vi "Dust Type Updater.vi"() -> ()   [LabVIEW 2013]
uses:
  <vilib>/Utility/miscctls.llb/LVPointTypeDef.ctl
  <vilib>/addons/database/Connection.llb/Conn Execute.vi
  <vilib>/addons/database/Recordset.llb/Rec Fetch Recordset Data (R).vi
  <vilib>/addons/database/Recordset.llb/Rec Destroy - Connection.vi
  <userlib>/_OpenG.lib/array/array.llb/Remove Duplicates from 1D Array (String)__ogtk.vi
  <userlib>/_OpenG.lib/array/array.llb/Search 1D Array (String)__ogtk.vi
  <userlib>/_OpenG.lib/array/array.llb/Index 1D Array Elements (I32)__ogtk.vi
  <userlib>/_OpenG.lib/array/array.llb/Search 1D Array (I32)__ogtk.vi
  <userlib>/_OpenG.lib/array/array.llb/Filter 1D Array (I32)__ogtk.vi
  <userlib>/_OpenG.lib/array/array.llb/Conditional Auto-Indexing Tunnel (I32)__ogtk.vi
  <userlib>/_OpenG.lib/comparison/comparison.llb/Boolean Changed__ogtk.vi
  <userlib>/_OpenG.lib/comparison/comparison.llb/String Changed__ogtk.vi
  <userlib>/_OpenG.lib/comparison/comparison.llb/U16 Changed__ogtk.vi
  <userlib>/_OpenG.lib/array/array.llb/Index 1D Array Elements (DBL)__ogtk.vi
  <vilib>/addons/database/_DB Variant To Data/Database Variant To Data.xnode
  <vilib>/addons/database/NI_Database_API.lvlib
panel:
  in  "Clear Errors?":bool
  out "Shoots":bool[](array[boolean])
  in  "Change Everything":bool
  in  "New Dust":T1 {"New Batch" min=1 max=3 step=1; "New Type" min=1 max=11 step=1}
  out "Bottle Weights":dbl[](array[numeric])
  in  "Updateable Properties":T2
  in  "Create New Entry":bool
  in  "Cancel":bool
  in  "Update":bool
  in  "Update current entry":bool
  out "error IO":errorcluster
  in  "stop":bool
  out "Comments":string[](array[string])
  out "Dust Names":string[](array[string])
  out "Dust Weights":dbl[](array[numeric])
  out "Sizes":string[](array[string])
  out "Typical Weights":dbl[](array[numeric])
  out "Densities":dbl[](array[numeric])
  out "Batch Nos":i32[](array[numeric])
  out "Dust Type":i32[](array[numeric])
  out "Dust Type Ids":i32[](array[numeric])
  out "Dust Properties":T3
  in  "Dust":T4 {"Batch" min=1 max=3 step=1; "Type" min=1 max=10 step=1}
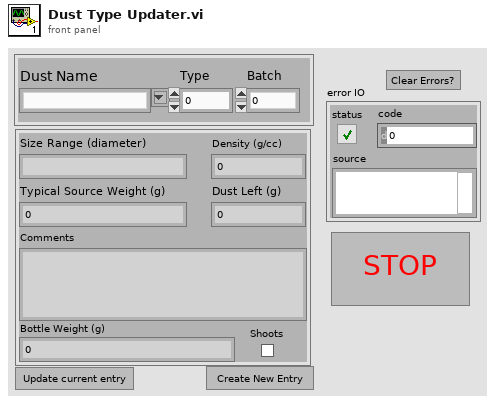
[diagram p1: front panel]
types:
  T1 = cluster{"New Dust Name":string, "New Type":u16, "New Batch":u16, "dust type id":u16, "Dust Left (g)":dbl, "Typical Source Weight (g)":dbl, "Density (g/cc)":dbl, "Size Range (diameter)":string, "Comments":string, "Bottle Weight (g)":dbl, "Shoots":bool}
  T2 = cluster{"Size Range (diameter)":string, "Density (g/cc)":dbl, "Typical Source Weight (g)":dbl, "Total Weight (g)":dbl, "Comments":string, "Bottle Weight (g)":dbl, "Shoots":bool}
  T3 = cluster{"Size Range (diameter)":string, "Density (g/cc)":dbl, "Typical Source Weight (g)":dbl, "Dust Left (g)":dbl, "Comments":string, "Bottle Weight (g)":dbl, "Shoots":bool}
  T4 = cluster{"Dust Name":string, "Type":u16, "Batch":u16, "dust type id":u16}
  T5 = typedef "LVPointTypeDef.ctl" = cluster{"Horizontal":i16, "Vertical":i16}
  T6 = enum8{"Enabled", "Disabled", "Disabled and Grayed Out"}
  T7 = typedef "NI_Database_API.lvlib/Conn ObjectReference.ctl" = refnum<k1>
  T8 = typedef "NI_Database_API.lvlib/Rec ObjectReference.ctl" = refnum<k1>
  T9 = cluster{"data":string, "data":dbl, "data":dbl, "data":dbl, "data":string, "data":dbl, "data":bool}
  T10 = cluster{"data":string, "data":dbl, "data":dbl, dbl, "data":string, "data":dbl, "data":bool}
  T11 = cluster{"Size Range (diameter)":string, "Density (g/cc)":dbl, "Typical Source Weight (g)":dbl, dbl, "Comments":string, "Bottle Weight (g)":dbl, "Shoots":bool}
  T12 = cluster{"Density (g/cc)":dbl, "Typical Source Weight (g)":dbl, "Size Range (diameter)":string, "Bottle Weight (g)":dbl, dbl, "Comments":string, i16}
  T13 = cluster{"dust type id":u16, "trimmed string":string, "New Type":u16, "New Batch":u16, "Density (g/cc)":dbl, "Typical Source Weight (g)":dbl, "Size Range (diameter)":string, "Bottle Weight (g)":dbl, "Dust Left (g)":dbl, "Comments":string, "Shoots":bool}
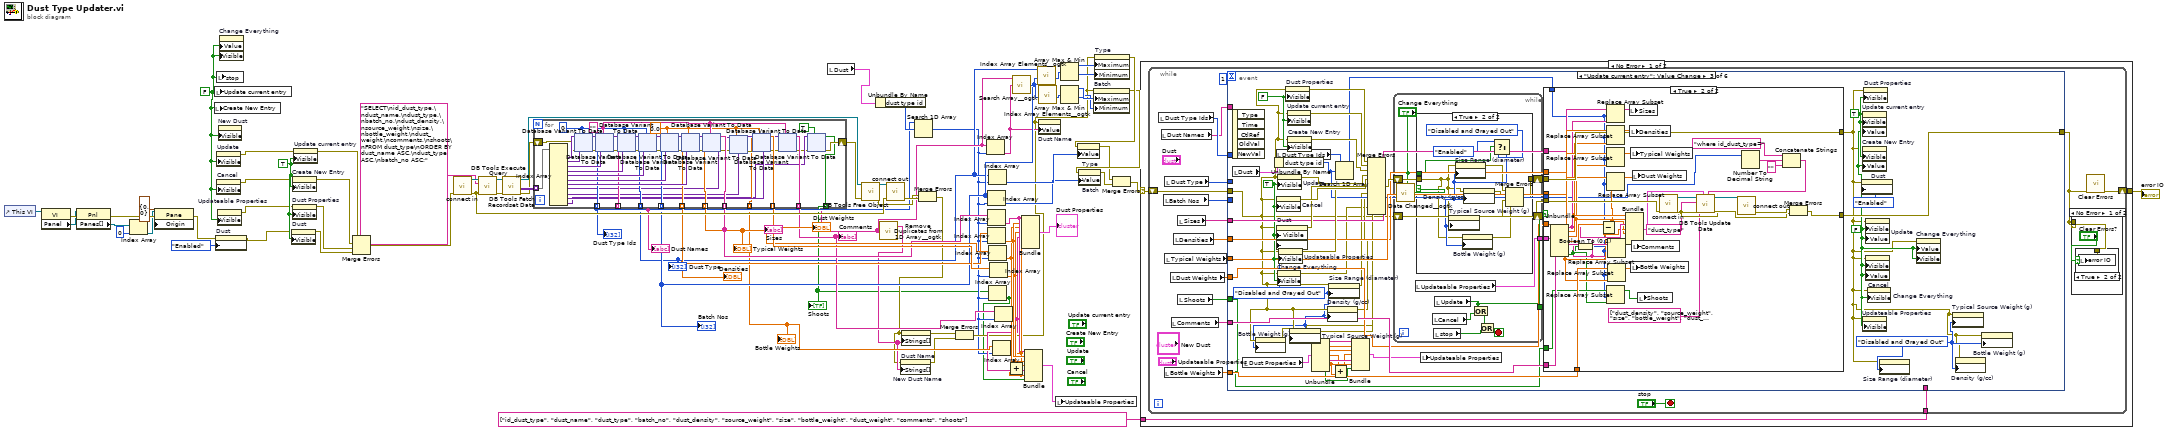
[diagram p0: block diagram]
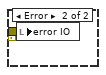
[diagram p3: hidden frame]
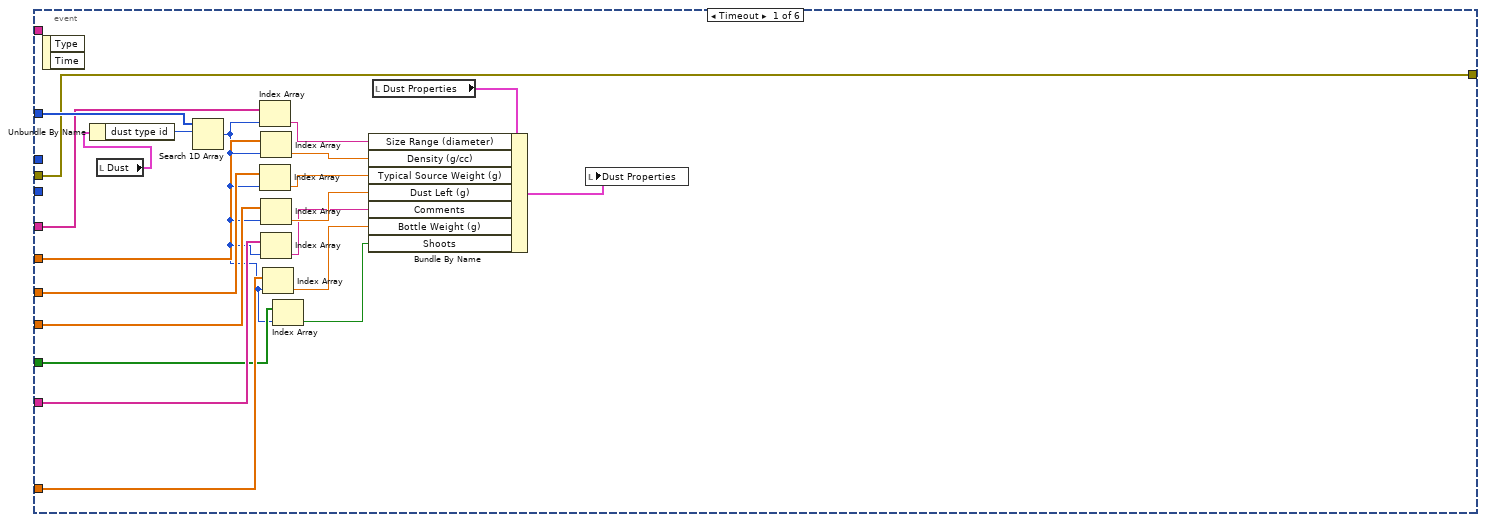
[diagram p4: hidden frame]
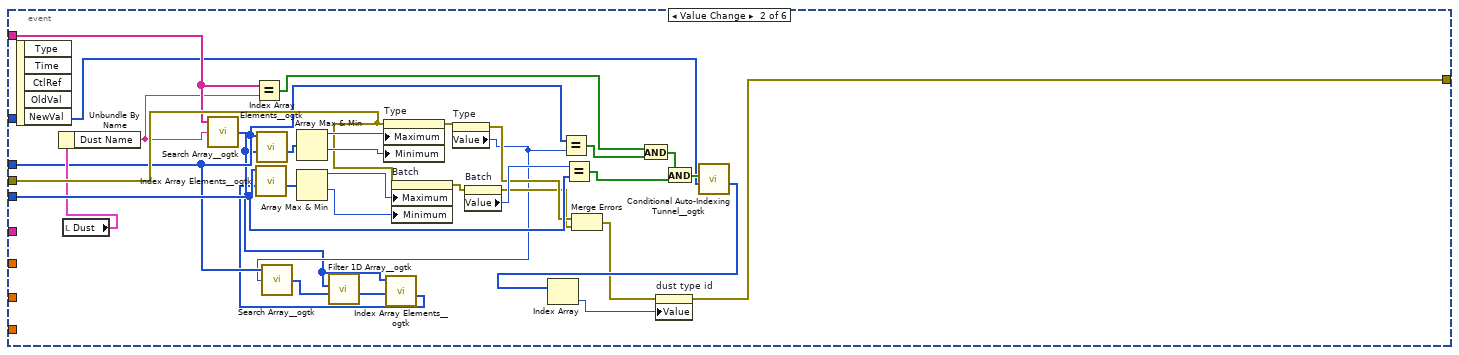
[diagram p5: hidden frame]
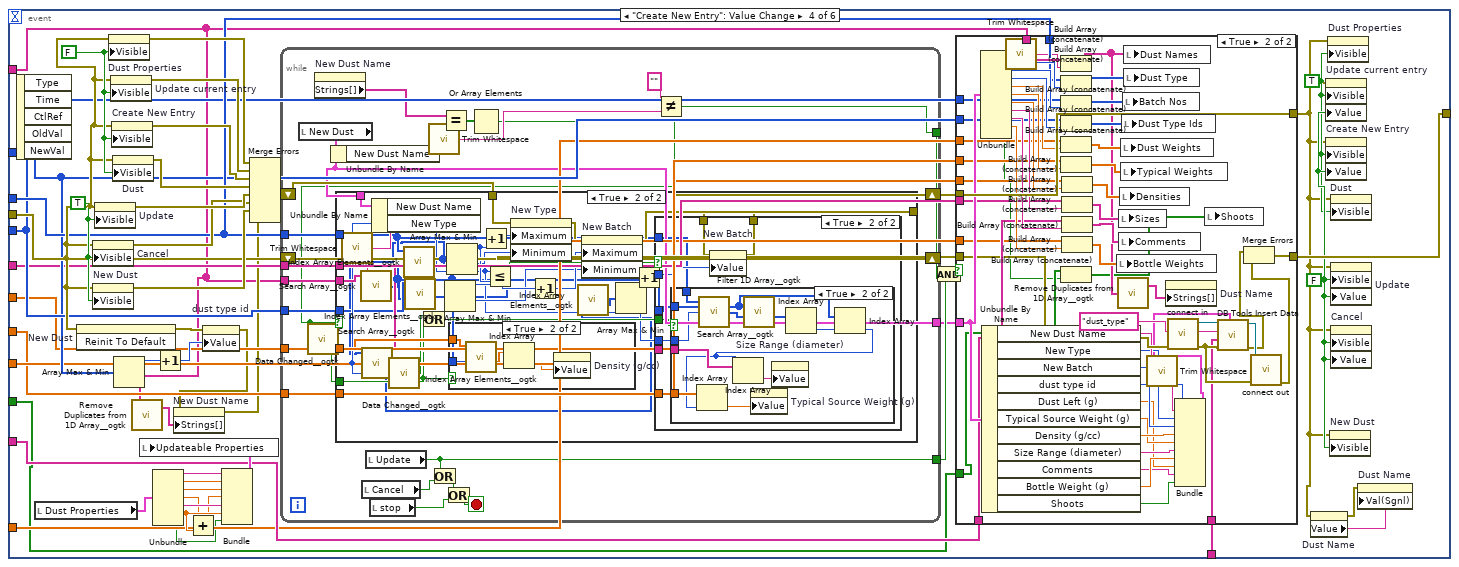
[diagram p8: hidden frame]
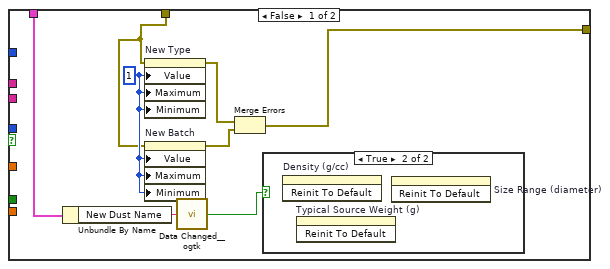
[diagram p10: hidden frame]
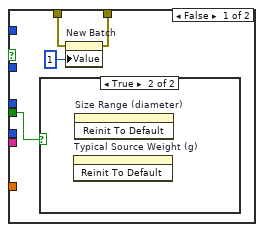
[diagram p13: hidden frame]
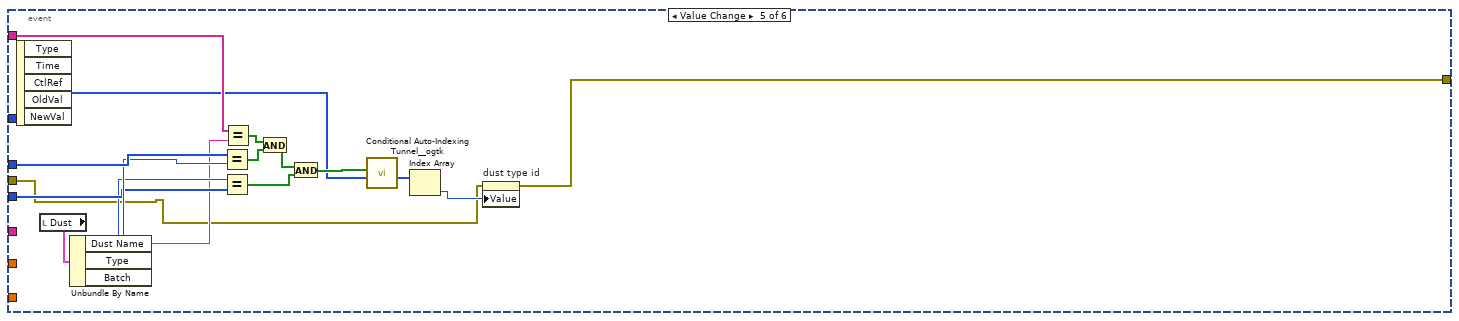
[diagram p16: hidden frame]
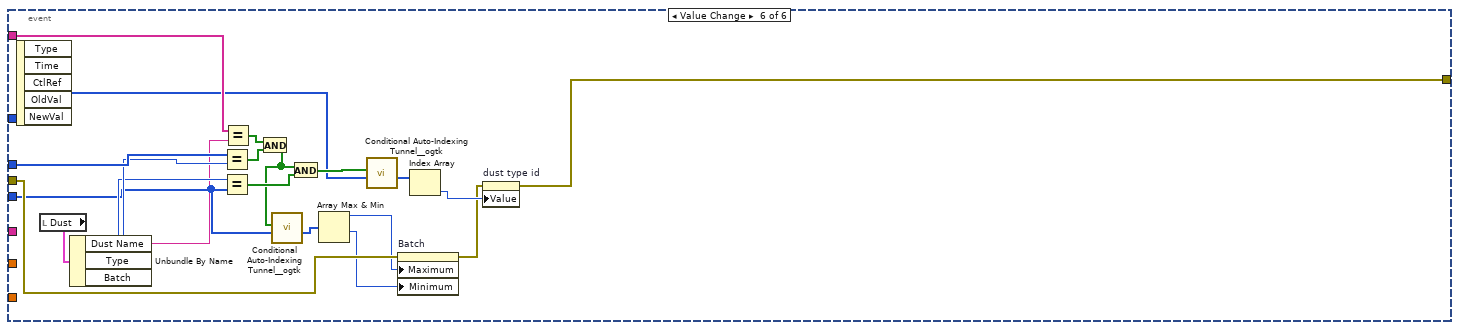
[diagram p17: hidden frame]
diagram:
  w40 = TRUE ("Visible")
  w13 = FALSE ("Update current entry")
  n1 = control-ref of="This VI"() -> (w9:refnum<vi>)
  n2 = property class="VI"(reference=w9) -> (error out=w8:errorcluster, "Panel"=w7:refnum<vi>)  [unwired: 1 in, 1 out]
  n3 = property class="Pnl"(reference=w7, error in=w8) -> (error out=w6:errorcluster, "Panes[]"=w5:refnum<vi>[])  [unwired: 1 out]
  n4 = Index Array(array=w5, index=0) -> (element=w3:refnum<vi>)
  n5 = property class="Pane"(reference=w3, error in=w6, "Origin"=T5 {"Horizontal"=0, "Vertical"=0}) -> (error out=w1:errorcluster)  [unwired: 1 out]
  n6 = local write "Create New Entry"(w13) -> ()
  n7 = local write "Update current entry"(w13) -> ()
  n8 = property on="Dust" class="Clust (strict)"(error in=w1, "DisabledEnum"=T6."Enabled" ("Disabled")) -> (error out=w31:errorcluster)  [unwired: 1 in, 1 out]
  n9 = local write "stop"(w13) -> ()
  n10 = property on="Update" class="Bool (strict)"("Visible"=w13) -> (error out=w37:errorcluster)  [unwired: 2 in, 1 out]
  n11 = property on="Cancel" class="Bool (strict)"("Visible"=w13) -> (error out=w38:errorcluster)  [unwired: 2 in, 1 out]
  n12 = property on="Updateable Properties" class="Clust (strict)"("Visible"=w13) -> (error out=w39:errorcluster)  [unwired: 2 in, 1 out]
  n13 = property on="New Dust" class="Clust (strict)"("Visible"=w13) -> ()  [unwired: 2 in, 2 out]
  n14 = property on="Change Everything" class="Bool (strict)"("Value"=w13, "Visible"=w13) -> ()  [unwired: 2 in, 2 out]
  n15 = property on="Dust" class="Clust (strict)"(error in=w31, "Visible"=w40) -> (error out=w32:errorcluster)  [unwired: 1 in, 1 out]
  n16 = property on="Create New Entry" class="Bool (strict)"(error in=w38, "Visible"=w40) -> (error out=w34:errorcluster)  [unwired: 1 in, 1 out]
  n17 = property on="Dust Properties" class="Clust (strict)"(error in=w39, "Visible"=w40) -> (error out=w33:errorcluster)  [unwired: 1 in, 1 out]
  n18 = property on="Update current entry" class="Bool (strict)"(error in=w37, "Visible"=w40) -> (error out=w35:errorcluster)  [unwired: 1 in, 1 out]
  n19 = Merge Errors(w35, w34, w33, w32) -> (w36:errorcluster)
  n20 = call <userlib>:"connect in.vi"("error in (no error)"=w36) -> ("error out"=w70:errorcluster, "Database Connection"=w77:T7)  [unwired: 7 in]
  n21 = call-poly <vilib>:"DB Tools Execute Query.vi"("error in (no error)"=w70, "SQL query"="SELECT\nid_dust_type,\ndust_name,\ndust_type,\nbatch_no,\ndust_density,\nsource_weight,\nsize,\nbottle_weight,\ndust_weight,\ncomments,\nshoots\nFROM dust_type\nORDER BY dust_name ASC,\ndust_type ASC,\nbatch_no ASC;", "connection reference"=w77) -> ("error out"=w79:errorcluster, "recordset reference"=w78:T8)  [unwired: 5 in]
  n22 = call-poly <vilib>:"DB Tools Fetch Recordset Data.vi"("error in (no error)"=w79, "recordset reference"=w78) -> ("error out"=w74:errorcluster, "recordset data"=w75:variant[][], "recordset reference out"=w71:T8)  [unwired: 3 in]
  n23 = for {
    tunnel: w75 -> [w118] mode=indexing
    shift-right: [w81] -> w72
    shift-left: w74 -> [w110]
    tunnel: [w102] -> w61 mode=indexing
    tunnel: [w101] -> w57 mode=indexing
    tunnel: [w100] -> w54 mode=indexing
    tunnel: [w99] -> w55 mode=indexing
    tunnel: [w98] -> w65 mode=indexing
    tunnel: [w97] -> w66 mode=indexing
    tunnel: [w96] -> w64 mode=indexing
    tunnel: [w95] -> w67 mode=indexing
    tunnel: [w92] -> w63 mode=indexing
    tunnel: [w85] -> w29 mode=indexing
    tunnel: [w80] -> w11 mode=indexing
    w88 = 0.0
    w94 = ""
    w103 = 0
    n24 = Index Array(array=w118) -> (element #1=w117:variant, element #2=w116:variant, element #3=w115:variant, element #4=w114:variant, element #5=w113:variant, element #6=w112:variant, element #7=w111:variant, element #8=w89:variant, element #9=w90:variant, element #10=w91:variant, element #11=w84:variant)  [unwired: 11 in]
    n25 = xnode "Database Variant To Data"("database variant"=w117, "error in (no error)"=w110, "type"=w103) -> ("data"=w102:i32, "error out"=w109:errorcluster)
    n26 = xnode "Database Variant To Data"("database variant"=w116, "error in (no error)"=w109, "type"=w94) -> ("data"=w101:string, "error out"=w108:errorcluster)
    n27 = xnode "Database Variant To Data"("database variant"=w115, "error in (no error)"=w108, "type"=w103) -> ("data"=w100:i32, "error out"=w107:errorcluster)
    n28 = xnode "Database Variant To Data"("database variant"=w114, "error in (no error)"=w107, "type"=w103) -> ("data"=w99:i32, "error out"=w106:errorcluster)
    n29 = xnode "Database Variant To Data"("database variant"=w113, "error in (no error)"=w106, "type"=w88) -> ("data"=w98:dbl, "error out"=w105:errorcluster)
    n30 = xnode "Database Variant To Data"("database variant"=w112, "error in (no error)"=w105, "type"=w88) -> ("data"=w97:dbl, "error out"=w104:errorcluster)
    n31 = xnode "Database Variant To Data"("database variant"=w111, "error in (no error)"=w104, "type"=w94) -> ("data"=w96:string, "error out"=w87:errorcluster)
    n32 = xnode "Database Variant To Data"("database variant"=w89, "error in (no error)"=w87, "type"=w88) -> ("data"=w85:dbl, "error out"=w86:errorcluster)
    n33 = xnode "Database Variant To Data"("database variant"=w90, "error in (no error)"=w86, "type"=w88) -> ("data"=w95:dbl, "error out"=w93:errorcluster)
    n34 = xnode "Database Variant To Data"("database variant"=w91, "error in (no error)"=w93, "type"=w94) -> ("data"=w92:string, "error out"=w82:errorcluster)
    n35 = xnode "Database Variant To Data"("database variant"=w84, "error in (no error)"=w82, "type"=TRUE) -> ("data"=w80:bool, "error out"=w81:errorcluster)
  }
  "Dust Type Ids" <- w61
  "Dust Type" <- w54
  "Batch Nos" <- w55
  "Densities" <- w65
  "Typical Weights" <- w66
  "Sizes" <- w64
  "Dust Weights" <- w67
  "Dust Names" <- w57
  "Comments" <- w63
  "Bottle Weights" <- w29
  "Shoots" <- w11
  n36 = local read "Dust"() -> (w41:T4)
  n37 = call-poly <vilib>:"DB Tools Free Object.vi"("error in (no error)"=w72, "recordset reference"=w71) -> ("error out"=w68:errorcluster, "connection reference"=w73:T7)  [unwired: 8 in]
  n38 = Unbundle By Name(w41) -> ("dust type id"=w62:u16)
  n39 = call-poly <userlib>:"Remove Duplicates from 1D Array__ogtk.vi"("Input Array"=w57) -> ("Output Array"=w18:string[])  [unwired: 1 out]
  n40 = call <userlib>:"connect out.vi"("error in (no error)"=w70, "connection reference"=w73) -> ("error out"=w69:errorcluster)  [unwired: 9 in]
  n41 = Search 1D Array(1D array=w61, element=w62) -> (index of element=w12:i32)  [unwired: 1 in]
  n42 = Merge Errors(w68, w69) -> (w17:errorcluster)
  n43 = property on="New Dust Name" class="CmbBox"(error in=w17, "Strings[]"=w18) -> (error out=w15:errorcluster)  [unwired: 1 in, 1 out]
  n44 = property on="Dust Name" class="CmbBox"(error in=w17, "Strings[]"=w18) -> (error out=w45:errorcluster)  [unwired: 1 in, 1 out]
  n45 = Merge Errors(w45, w15) -> (w16:errorcluster)
  n46 = Index Array(array=w57, index=w12) -> (element=w19:string)
  n47 = Index Array(array=w64, index=w12) -> (element=w26:string)
  n48 = Index Array(array=w65, index=w12) -> (element=w25:dbl)
  n49 = Index Array(array=w55, index=w12) -> (element=w58:i32)
  n50 = Index Array(array=w11, index=w12) -> (element=w10:bool)
  n51 = Index Array(array=w54, index=w12) -> (element=w59:i32)
  n52 = Index Array(array=w66, index=w12) -> (element=w24:dbl)
  n53 = Index Array(array=w67, index=w12) -> (element=w23:dbl)
  n54 = Index Array(array=w29, index=w12) -> (element=w20:dbl)
  n55 = Index Array(array=w63, index=w12) -> (element=w22:string)
  n56 = Add(x=w23, y=w20) -> (x+y=w21:dbl)
  n57 = call-poly <userlib>:"Search Array__ogtk.vi"("Array"=w57, "Element Data"=w19) -> ("Indices of Elements"=w56:i32[])  [unwired: 7 in]
  n58 = Bundle("data"=w26, "data"=w25, "data"=w24, "data"=w23, "data"=w22, "data"=w20, "data"=w10) -> (→"Dust Properties":T9)  [unwired: 1 in]
  n59 = Bundle("data"=w26, "data"=w25, "data"=w24, w21, "data"=w22, "data"=w20, "data"=w10) -> (w27:T10)  [unwired: 1 in]
  n60 = call-poly <userlib>:"Index Array Elements__ogtk.vi"("indices"=w56, "array"=w54) -> ("elements"=w53:i32[])  [unwired: 9 in]
  n61 = call-poly <userlib>:"Index Array Elements__ogtk.vi"("indices"=w56, "array"=w55) -> ("elements"=w52:i32[])  [unwired: 9 in]
  n62 = property on="Dust Name" class="CmbBox"(error in=w16, "Value"=w19) -> ()  [unwired: 1 in, 2 out]
  n63 = local write "Updateable Properties"(w27) -> ()
  n64 = Array Max & Min(array=w53) -> (max value=w51:i32, min value=w50:i32)  [unwired: 2 out]
  n65 = Array Max & Min(array=w52) -> (max value=w49:i32, min value=w48:i32)  [unwired: 2 out]
  n66 = property on="Batch" class="DigNum (strict)"(error in=w16, "Maximum"=w49, "Minimum"=w48) -> (error out=w46:errorcluster)  [unwired: 1 in, 1 out]
  n67 = property on="Batch" class="DigNum (strict)"(error in=w46, "Value"=w58) -> (error out=w43:errorcluster)  [unwired: 1 in, 1 out]
  n68 = property on="Type" class="DigNum (strict)"(error in=w16, "Maximum"=w51, "Minimum"=w50) -> (error out=w47:errorcluster)  [unwired: 1 in, 1 out]
  n69 = property on="Type" class="DigNum (strict)"(error in=w47, "Value"=w59) -> (error out=w44:errorcluster)  [unwired: 1 in, 1 out]
  n70 = Merge Errors(w44, w43) -> (w42:errorcluster)
  n71 = case shown="No Error" w42 {
    selector: w42 -> [w473 w901]
    tunnel: [w472 w901] -> w60
    tunnel: string[] ["id_dust_type", "dust_name", "dust_type", "batch_no", "dust_density", "source_weight", "size", "bottle_weight", "dust_weight", "comments", "shoots"] ("columns") -> [w471 _]
    frame No Error {
      n72 = while {
        shift-right: [w479] -> w472
        shift-left: w473 -> [w483]
        tunnel: w471 -> [w476]
        stop <- "stop" stop-if-true
        n73 = local read "Dust Type Ids"() -> (w489:i32[])
        n74 = local read "Dust Names"() -> (w482:string[])
        n75 = local read "Batch Nos"() -> (w480:i32[])
        n76 = local read "Bottle Weights"() -> (w477:dbl[])
        n77 = local read "Dust Type"() -> (w481:i32[])
        n78 = local read "Typical Weights"() -> (w486:dbl[])
        n79 = local read "Dust Weights"() -> (w485:dbl[])
        n80 = local read "Comments"() -> (w484:string[])
        n81 = local read "Densities"() -> (w487:dbl[])
        n82 = local read "Sizes"() -> (w488:string[])
        n83 = local read "Shoots"() -> (w475:bool[])
        n84 = event shown="[2] \"Update current entry\": Value Change" {
          selector: _ -> [_ _ _ _ _ _]
          dyn-events: _ -> [_ _ _ _ _ _]
          timeout: 1 -> [_ _ _ _ _ _]
          tunnel: w489 -> [w514 w532 _ w679 w869 w892]
          tunnel: w488 -> [w513 _ w567 w675 _ _]
          tunnel: w487 -> [w512 _ w568 w676 _ _]
          tunnel: w486 -> [w511 _ w569 w677 _ _]
          tunnel: w485 -> [w510 _ w570 w678 _ _]
          tunnel: w484 -> [w509 _ w571 w674 _ _]
          tunnel: w483 -> [w501 w543 w557 w685 w863 w886]
          tunnel: [w501 w526 w575 w699 w866 w889] -> w474
          tunnel: w482 -> [_ w540 _ w670 w879 w900]
          tunnel: w481 -> [_ w521 _ w681 w878 w899]
          tunnel: w480 -> [_ w539 _ w680 w876 w883]
          tunnel: w477 -> [w499 _ w572 w673 _ _]
          tunnel: w476 -> [_ _ _ w668 _ _]
          tunnel: w475 -> [w497 _ w548 w662 _ _]
          event Timeout {
            n85 = event-data() -> ()  [unwired: 1 in, 2 out]
            n86 = local read "Dust"() -> (w500:T4)
            n87 = Unbundle By Name(w500) -> ("dust type id"=w515:u16)
            n88 = Search 1D Array(1D array=w514, element=w515) -> (index of element=w496:i32)  [unwired: 1 in]
            n89 = Index Array(array=w513, index=w496) -> (element=w508:string)
            n90 = Index Array(array=w511, index=w496) -> (element=w506:dbl)
            n91 = Index Array(array=w512, index=w496) -> (element=w507:dbl)
            n92 = Index Array(array=w510, index=w496) -> (element=w505:dbl)
            n93 = Index Array(array=w509, index=w496) -> (element=w504:string)
            n94 = Index Array(array=w499, index=w496) -> (element=w498:dbl)
            n95 = Index Array(array=w497, index=w496) -> (element=w495:bool)
            n96 = local read "Dust Properties"() -> (w502:T3)
            n97 = Bundle By Name(cluster=w502, "Size Range (diameter)"=w508, "Density (g/cc)"=w507, "Typical Source Weight (g)"=w506, "Dust Left (g)"=w505, "Comments"=w504, "Bottle Weight (g)"=w498, "Shoots"=w495) -> (w503:T3)
            n98 = local write "Dust Properties"(w503) -> ()
          }
          event "Dust.Dust Name": Value Change {
            n99 = event-data() -> ()  [unwired: 1 in, 5 out]
            n100 = local read "Dust"() -> (w525:T4)
            n101 = Unbundle By Name(w525) -> ("Dust Name"=w522:string)
            n102 = call-poly <userlib>:"Search Array__ogtk.vi"("Array"=w540, "Element Data"=w522) -> ("Indices of Elements"=w517:i32[])  [unwired: 7 in]
            n103 = Equal?(x=w540, y=w522) -> (x = y?=w536:bool[])
            n104 = call-poly <userlib>:"Index Array Elements__ogtk.vi"("indices"=w517, "array"=w521) -> ("elements"=w547:i32[])  [unwired: 9 in]
            n105 = Array Max & Min(array=w547) -> (max value=w545:i32, min value=w544:i32)  [unwired: 2 out]
            n106 = property on="Type" class="DigNum (strict)"(error in=w543, "Maximum"=w545, "Minimum"=w544) -> (error out=w541:errorcluster)  [unwired: 1 in, 1 out]
            n107 = property on="Type" class="DigNum (strict)"(error in=w541) -> (error out=w529:errorcluster, "Value"=w520:u16)  [unwired: 1 in, 1 out]
            n108 = call-poly <userlib>:"Search Array__ogtk.vi"("Array"=w521, "Element Data"=w520) -> ("Indices of Elements"=w519:i32[])  [unwired: 7 in]
            n109 = call-poly <userlib>:"Filter 1D Array__ogtk.vi"("items to filter"=w519, "array"=w517) -> ("filtered item indices"=w518:i32[])  [unwired: 4 in, 1 out]
            n110 = call-poly <userlib>:"Index Array Elements__ogtk.vi"("indices"=w518, "array"=w517) -> ("elements"=w516:i32[])  [unwired: 9 in]
            n111 = call-poly <userlib>:"Index Array Elements__ogtk.vi"("indices"=w516, "array"=w539) -> ("elements"=w546:i32[])  [unwired: 9 in]
            n112 = Array Max & Min(array=w546) -> (max value=w523:i32, min value=w524:i32)  [unwired: 2 out]
            n113 = property on="Batch" class="DigNum (strict)"(error in=w543, "Maximum"=w523, "Minimum"=w524) -> (error out=w542:errorcluster)  [unwired: 1 in, 1 out]
            n114 = property on="Batch" class="DigNum (strict)"(error in=w542) -> (error out=w528:errorcluster, "Value"=w538:u16)  [unwired: 1 in, 1 out]
            n115 = Equal?(x=w521, y=w520) -> (x = y?=w537:bool[])
            n116 = Equal?(x=w538, y=w539) -> (x = y?=w534:bool[])
            n117 = Merge Errors(w529, w528) -> (w527:errorcluster)
            n118 = And(x=w536, y=w537) -> (x .and. y?=w535:bool[])
            n119 = And(x=w535, y=w534) -> (x .and. y?=w533:bool[])
            n120 = call-poly <userlib>:"Conditional Auto-Indexing Tunnel__ogtk.vi"("Array in"=w532, "Elements to keep"=w533) -> ("Filtered Array out"=w531:i32[])  [unwired: 5 in]
            n121 = Index Array(array=w531) -> (element=w530:i32)  [unwired: 1 in]
            n122 = property on="dust type id" class="Ring (strict)"(error in=w527, "Value"=w530) -> (error out=w526:errorcluster)  [unwired: 1 in, 1 out]
          }
          event "Update current entry": Value Change {
            w555 = T6."Disabled and Grayed Out" ("Disabled")
            w552 = T6."Disabled and Grayed Out" ("Disabled")
            w554 = FALSE ("Visible")
            w577 = TRUE ("Visible")
            w559 = TRUE ("Visible")
            w580 = FALSE ("Update current entry")
            n123 = event-data() -> ()  [unwired: 1 in, 5 out]
            n124 = local read "Dust"() -> (w591:T4)
            n125 = local read "Dust Properties"() -> (w551:T3)
            n126 = property on="Bottle Weight (g)" class="DigNum (strict)"(error in=w557, "DisabledEnum"=w552) -> (error out=w556:errorcluster)  [unwired: 1 in, 1 out]
            n127 = Unbundle By Name(w591) -> ("dust type id"=w563:u16)
            n128 = local read "Dust Type Ids"() -> (w590:i32[])
            n129 = property on="Cancel" class="Bool (strict)"(error in=w557, "Visible"=w559) -> (error out=w586:errorcluster)  [unwired: 1 in, 1 out]
            n130 = property on="Dust" class="Clust (strict)"(error in=w557, "Visible"=w559, "DisabledEnum"=w552) -> (error out=w585:errorcluster)  [unwired: 1 in, 1 out]
            n131 = property on="Change Everything" class="Bool (strict)"(error in=w557, "Visible"=w559) -> (error out=w558:errorcluster)  [unwired: 1 in, 1 out]
            n132 = property on="Update" class="Bool (strict)"(error in=w557, "Visible"=w559) -> (error out=w587:errorcluster)  [unwired: 1 in, 1 out]
            n133 = property on="Updateable Properties" class="Clust (strict)"(error in=w557, "Visible"=w559) -> (error out=w584:errorcluster)  [unwired: 1 in, 1 out]
            n134 = property on="Dust Properties" class="Clust (strict)"(error in=w557, "Visible"=w580) -> (error out=w579:errorcluster)  [unwired: 1 in, 1 out]
            n135 = property on="Update current entry" class="Bool (strict)"(error in=w557, "Visible"=w580) -> (error out=w589:errorcluster)  [unwired: 1 in, 1 out]
            n136 = property on="Create New Entry" class="Bool (strict)"(error in=w557, "Visible"=w580) -> (error out=w588:errorcluster)  [unwired: 1 in, 1 out]
            n137 = property on="Typical Source Weight (g)" class="DigNum (strict)"(error in=w557, "DisabledEnum"=w552) -> (error out=w560:errorcluster)  [unwired: 1 in, 1 out]
            n138 = Unbundle(w551) -> ("Size Range (diameter)"=w595:string, "Density (g/cc)"=w594:dbl, "Typical Source Weight (g)"=w593:dbl, "Dust Left (g)"=w565:dbl, "Comments"=w592:string, "Bottle Weight (g)"=w566:dbl, "Shoots"=w549:bool)
            n139 = property on="Density (g/cc)" class="DigNum (strict)"(error in=w557, "DisabledEnum"=w552) -> (error out=w561:errorcluster)  [unwired: 1 in, 1 out]
            n140 = property on="Size Range (diameter)" class="Str"(error in=w557, "DisabledEnum"=w552) -> (error out=w562:errorcluster)  [unwired: 1 in, 1 out]
            n141 = Add(x=w565, y=w566) -> (x+y=w564:dbl)
            n142 = Search 1D Array(1D array=w590, element=w563) -> (index of element=w574:i32)  [unwired: 1 in]
            n143 = Bundle("Size Range (diameter)"=w595, "Density (g/cc)"=w594, "Typical Source Weight (g)"=w593, w564, "Comments"=w592, "Bottle Weight (g)"=w566, "Shoots"=w549) -> (w550:T11)  [unwired: 1 in]
            n144 = Merge Errors(w579, w589, w588, w587, w586, w585, w584, w562, w561, w560, w558, w556) -> (w583:errorcluster)
            n145 = while {
              shift-right: [w639] -> w581
              shift-left: w583 -> [w643]
              tunnel: [w649] -> w573
              tunnel: [w647] -> w582
              shift-right: [w642] -> w576
              shift-left: w557 -> [w642]
              stop <- w645 stop-if-true
              n146 = call-poly <userlib>:"Data Changed__ogtk.vi"("Boolean"="Change Everything") -> ("Changed"=w641:bool)
              n147 = local read "Updateable Properties"() -> (w649:T2)
              n148 = case shown="True" w641 {
                tunnel: w643 -> [w650 w656]
                tunnel: "Change Everything" -> [_ w660]
                tunnel: [w650 w651] -> w639
                frame False {
                }
                frame True {
                  n149 = Select(t=T6."Enabled" ("Disabled"), s=w660, f=T6."Disabled and Grayed Out" ("Disabled")) -> (s? t:f=w657:T6)
                  n150 = property on="Typical Source Weight (g)" class="DigNum (strict)"(error in=w656, "DisabledEnum"=w657) -> (error out=w653:errorcluster)  [unwired: 1 in, 1 out]
                  n151 = property on="Size Range (diameter)" class="Str"(error in=w656, "DisabledEnum"=w657) -> (error out=w655:errorcluster)  [unwired: 1 in, 1 out]
                  n152 = property on="Bottle Weight (g)" class="DigNum (strict)"(error in=w656, "DisabledEnum"=w657) -> (error out=w652:errorcluster)  [unwired: 1 in, 1 out]
                  n153 = property on="Density (g/cc)" class="DigNum (strict)"(error in=w656, "DisabledEnum"=w657) -> (error out=w654:errorcluster)  [unwired: 1 in, 1 out]
                  n154 = Merge Errors(w655, w654, w653, w652) -> (w651:errorcluster)
                }
              }
              n155 = local read "Cancel"() -> (w646:bool)
              n156 = local read "stop"() -> (w644:bool)
              n157 = local read "Update"() -> (w647:bool)
              n158 = Or(x=w647, y=w646) -> (x .or. y?=w648:bool)
              n159 = Or(x=w648, y=w644) -> (x .or. y?=w645:bool)
            }
            n160 = local write "Updateable Properties"(w550) -> ()
            n161 = case shown="True" w582 {
              tunnel: w581 -> [w597 w638]
              tunnel: [w597 w638] -> w553
              tunnel: w576 -> [w596 w623]
              tunnel: [w596 w622] -> w575
              tunnel: w574 -> [_ w600]
              tunnel: w573 -> [_ w637]
              tunnel: w572 -> [_ w636]
              tunnel: w571 -> [_ w635]
              tunnel: w570 -> [_ w634]
              tunnel: w569 -> [_ w633]
              tunnel: w568 -> [_ w632]
              tunnel: w567 -> [_ w631]
              tunnel: w563 -> [_ w603]
              tunnel: w548 -> [_ w601]
              frame False {
              }
              frame True {
                n162 = Unbundle(w637) -> ("Size Range (diameter)"=w608:string, "Density (g/cc)"=w610:dbl, "Typical Source Weight (g)"=w609:dbl, "Total Weight (g)"=w624:dbl, "Comments"=w605:string, "Bottle Weight (g)"=w607:dbl, "Shoots"=w599:bool)
                n163 = Boolean To (0,1)(Boolean=w599) -> (0, 1=w602:i16)
                n164 = Subtract(x=w624, y=w607) -> (x-y=w606:dbl)
                n165 = Replace Array Subset(array=w631, new element=w608, index=w600) -> (w630:string[])
                n166 = Replace Array Subset(array=w632, new element=w610, index=w600) -> (w629:dbl[])
                n167 = Replace Array Subset(array=w633, new element=w609, index=w600) -> (w628:dbl[])
                n168 = Replace Array Subset(array=w634, new element=w606, index=w600) -> (w627:dbl[])
                n169 = Replace Array Subset(array=w601, new element=w599, index=w600) -> (w598:bool[])
                n170 = Replace Array Subset(array=w636, new element=w607, index=w600) -> (w626:dbl[])
                n171 = Replace Array Subset(array=w635, new element=w605, index=w600) -> (w625:string[])
                n172 = Bundle("Density (g/cc)"=w610, "Typical Source Weight (g)"=w609, "Size Range (diameter)"=w608, "Bottle Weight (g)"=w607, w606, "Comments"=w605, w602) -> (w604:T12)  [unwired: 1 in]
                n173 = local write "Sizes"(w630) -> ()
                n174 = local write "Densities"(w629) -> ()
                n175 = local write "Typical Weights"(w628) -> ()
                n176 = local write "Bottle Weights"(w626) -> ()
                n177 = local write "Comments"(w625) -> ()
                n178 = local write "Dust Weights"(w627) -> ()
                n179 = local write "Shoots"(w598) -> ()
                n180 = call <userlib>:"connect in.vi"("error in (no error)"=w623) -> ("error out"=w619:errorcluster, "Database Connection"=w617:T7)  [unwired: 7 in]
                n181 = Number To Decimal String(number=w603) -> (decimal integer string=w613:string)  [unwired: 1 in]
                n182 = Concatenate Strings("where id_dust_type=" ("condition"), w613, "" ("string")) -> (w611:string)
                n183 = call <vilib>:"DB Tools Update Data.vi"("condition"=w611, "data"=w604, "error in (no error)"=w619, "columns"=string[] ["dust_density", "source_weight", "size", "bottle_weight", "dust_weight", "comments", "shoots"], "table"="dust_type", "connection reference"=w617) -> ("error out"=w620:errorcluster, "connection reference out"=w616:T7)  [unwired: 4 in]
                n184 = call <userlib>:"connect out.vi"("error in (no error)"=w619, "connection reference"=w616) -> ("error out"=w621:errorcluster)  [unwired: 9 in]
                n185 = Merge Errors(w621, w620) -> (w622:errorcluster)
              }
            }
            n186 = property on="Dust" class="Clust (strict)"(error in=w553, "DisabledEnum"=T6."Enabled" ("Disabled")) -> ()  [unwired: 1 in, 2 out]
            n187 = property on="Update current entry" class="Bool (strict)"(error in=w553, "Visible"=w577, "Value"=w554) -> ()  [unwired: 1 in, 2 out]
            n188 = property on="Create New Entry" class="Bool (strict)"(error in=w553, "Visible"=w577, "Value"=w554) -> ()  [unwired: 1 in, 2 out]
            n189 = property on="Updateable Properties" class="Clust (strict)"(error in=w553, "Visible"=w554) -> ()  [unwired: 1 in, 2 out]
            n190 = property on="Dust Properties" class="Clust (strict)"(error in=w553, "Visible"=w577) -> ()  [unwired: 1 in, 2 out]
            n191 = property on="Update" class="Bool (strict)"(error in=w553, "Visible"=w554, "Value"=w554) -> ()  [unwired: 1 in, 2 out]
            n192 = property on="Cancel" class="Bool (strict)"(error in=w553, "Visible"=w554, "Value"=w554) -> ()  [unwired: 1 in, 2 out]
            n193 = property on="Change Everything" class="Bool (strict)"(error in=w553, "Visible"=w554) -> ()  [unwired: 1 in, 2 out]
            n194 = property on="Size Range (diameter)" class="Str"(error in=w553, "DisabledEnum"=w555) -> ()  [unwired: 1 in, 2 out]
            n195 = property on="Change Everything" class="Bool (strict)"(error in=w553, "Value"=w554, "Visible"=w554) -> ()  [unwired: 1 in, 2 out]
            n196 = property on="Typical Source Weight (g)" class="DigNum (strict)"(error in=w553, "DisabledEnum"=w555) -> ()  [unwired: 1 in, 2 out]
            n197 = property on="Density (g/cc)" class="DigNum (strict)"(error in=w553, "DisabledEnum"=w555) -> ()  [unwired: 1 in, 2 out]
            n198 = property on="Bottle Weight (g)" class="DigNum (strict)"(error in=w553, "DisabledEnum"=w555) -> ()  [unwired: 1 in, 2 out]
          }
          event "Create New Entry": Value Change {
            w688 = FALSE ("Visible")
            w687 = TRUE ("Visible")
            w693 = TRUE ("Visible")
            w694 = FALSE ("Update current entry")
            n199 = event-data() -> ()  [unwired: 1 in, 5 out]
            n200 = local read "Dust Properties"() -> (w711:T3)
            n201 = invoke on="New Dust" class="Clust (strict)" method="Reinit To Default"(error in=w685) -> (error out=w684:errorcluster)  [unwired: 2 in, 2 out]
            n202 = property on="Cancel" class="Bool (strict)"(error in=w685, "Visible"=w693) -> (error out=w690:errorcluster)  [unwired: 1 in, 1 out]
            n203 = property on="New Dust" class="Clust (strict)"(error in=w685, "Visible"=w693) -> (error out=w689:errorcluster)  [unwired: 1 in, 1 out]
            n204 = property on="Update" class="Bool (strict)"(error in=w685, "Visible"=w693) -> (error out=w691:errorcluster)  [unwired: 1 in, 1 out]
            n205 = property on="Dust Properties" class="Clust (strict)"(error in=w685, "Visible"=w694) -> (error out=w701:errorcluster)  [unwired: 1 in, 1 out]
            n206 = property on="Update current entry" class="Bool (strict)"(error in=w685, "Visible"=w694) -> (error out=w706:errorcluster)  [unwired: 1 in, 1 out]
            n207 = property on="Create New Entry" class="Bool (strict)"(error in=w685, "Visible"=w694) -> (error out=w705:errorcluster)  [unwired: 1 in, 1 out]
            n208 = property on="Dust" class="Clust (strict)"(error in=w685, "Visible"=w694) -> (error out=w692:errorcluster)  [unwired: 1 in, 1 out]
            n209 = Array Max & Min(array=w679) -> (max value=w683:i32)  [unwired: 3 out]
            n210 = call-poly <userlib>:"Remove Duplicates from 1D Array__ogtk.vi"("Input Array"=w670) -> ("Output Array"=w669:string[])  [unwired: 1 out]
            n211 = Unbundle(w711) -> ("Size Range (diameter)"=w710:string, "Density (g/cc)"=w709:dbl, "Typical Source Weight (g)"=w708:dbl, "Dust Left (g)"=w696:dbl, "Comments"=w707:string, "Bottle Weight (g)"=w697:dbl, "Shoots"=w661:bool)
            n212 = Increment(x=w683) -> (x+1=w682:i32)
            n213 = Add(x=w696, y=w697) -> (x+y=w695:dbl)
            n214 = property on="dust type id" class="DigNum (strict)"(error in=w684, "Value"=w682) -> (error out=w672:errorcluster)  [unwired: 1 in, 1 out]
            n215 = property on="New Dust Name" class="CmbBox"(error in=w672, "Strings[]"=w669) -> (error out=w671:errorcluster)  [unwired: 1 in, 1 out]
            n216 = Bundle("Size Range (diameter)"=w710, "Density (g/cc)"=w709, "Typical Source Weight (g)"=w708, w695, "Comments"=w707, "Bottle Weight (g)"=w697, "Shoots"=w661) -> (w698:T11)  [unwired: 1 in]
            n217 = local write "Updateable Properties"(w698) -> ()
            n218 = Merge Errors(w701, w706, w705, w692, w691, w690, w689, w671) -> (w704:errorcluster)
            n219 = while {
              shift-right: [w782] -> w702
              shift-left: w704 -> [w783]
              tunnel: [w792] -> w703
              shift-right: [w793] -> w700
              shift-left: w685 -> [w793]
              tunnel: [w780] -> w686
              tunnel: w670 -> [w786]
              tunnel: w680 -> [w785]
              tunnel: w681 -> [w784]
              tunnel: w676 -> [w781]
              tunnel: w675 -> [w779]
              tunnel: w677 -> [w778]
              tunnel: [w776] -> w666
              stop <- w791 stop-if-true
              n220 = local read "New Dust"() -> (w780:T1)
              n221 = property on="New Dust Name" class="CmbBox"() -> ("Strings[]"=w789:string[])  [unwired: 2 in, 2 out]
              n222 = Unbundle By Name(w780) -> ("New Dust Name"=w787:string)
              n223 = local read "Cancel"() -> (w795:bool)
              n224 = local read "Update"() -> (w792:bool)
              n225 = local read "stop"() -> (w790:bool)
              n226 = call <vilib>:"Trim Whitespace.vi"("string"=w787) -> ("trimmed string"=w775:string)  [unwired: 1 in]
              n227 = Or(x=w792, y=w795) -> (x .or. y?=w794:bool)
              n228 = Equal?(x=w789, y=w775) -> (x = y?=w788:bool[])
              n229 = Or(x=w794, y=w790) -> (x .or. y?=w791:bool)
              n230 = Or Array Elements(Boolean array=w788) -> (logical OR=w774:bool)
              n231 = call-poly <userlib>:"Data Changed__ogtk.vi"("Boolean"=w774) -> ("Changed"=w773:bool)
              n232 = case shown="True" w774 {
                tunnel: w786 -> [_ w834]
                tunnel: w785 -> [_ w811]
                tunnel: w784 -> [_ w813]
                tunnel: w783 -> [w802 w830]
                tunnel: [w799 w831] -> w782
                tunnel: w781 -> [_ w822]
                tunnel: w780 -> [w798 w824]
                tunnel: w779 -> [_ w820]
                tunnel: w778 -> [_ w819]
                tunnel: w773 -> [_ w814]
                frame False {
                  w803 = u16 1 ("Value")
                  n233 = Unbundle By Name(w798) -> ("New Dust Name"=w797:string)
                  n234 = property on="New Type" class="DigNum (strict)"(error in=w802, "Value"=w803, "Maximum"=w803, "Minimum"=w803) -> (error out=w801:errorcluster)  [unwired: 1 in, 1 out]
                  n235 = property on="New Batch" class="DigNum (strict)"(error in=w802, "Value"=w803, "Maximum"=w803, "Minimum"=w803) -> (error out=w800:errorcluster)  [unwired: 1 in, 1 out]
                  n236 = call-poly <userlib>:"Data Changed__ogtk.vi"("String"=w797) -> ("Changed"=w796:bool)
                  n237 = Merge Errors(w801, w800) -> (w799:errorcluster)
                  n238 = case shown="True" w796 {
                    frame False {
                    }
                    frame True {
                      n239 = invoke on="Density (g/cc)" class="DigNum (strict)" method="Reinit To Default"() -> ()  [unwired: 3 in, 3 out]
                      n240 = invoke on="Typical Source Weight (g)" class="DigNum (strict)" method="Reinit To Default"() -> ()  [unwired: 3 in, 3 out]
                      n241 = invoke on="Size Range (diameter)" class="Str" method="Reinit To Default"() -> ()  [unwired: 3 in, 3 out]
                    }
                  }
                }
                frame True {
                  n242 = Unbundle By Name(w824) -> ("New Dust Name"=w823:string, "New Type"=w812:u16)
                  n243 = call <vilib>:"Trim Whitespace.vi"("string"=w823) -> ("trimmed string"=w816:string)  [unwired: 1 in]
                  n244 = call-poly <userlib>:"Search Array__ogtk.vi"("Array"=w834, "Element Data"=w816) -> ("Indices of Elements"=w808:i32[])  [unwired: 7 in]
                  n245 = call-poly <userlib>:"Data Changed__ogtk.vi"("U16"=w812) -> ("Changed"=w821:bool)
                  n246 = call-poly <userlib>:"Index Array Elements__ogtk.vi"("indices"=w808, "array"=w813) -> ("elements"=w810:i32[])  [unwired: 9 in]
                  n247 = call-poly <userlib>:"Search Array__ogtk.vi"("Array"=w810, "Element Data"=w812) -> ("Indices of Elements"=w809:i32[])  [unwired: 7 in]
                  n248 = call-poly <userlib>:"Index Array Elements__ogtk.vi"("indices"=w808, "array"=w811) -> ("elements"=w804:i32[])  [unwired: 9 in]
                  n249 = Or(x=w821, y=w814) -> (x .or. y?=w815:bool)
                  n250 = Array Max & Min(array=w804) -> (max value=w832:i32, min value=w817:i32)  [unwired: 2 out]
                  n251 = Array Max & Min(array=w810) -> (max value=w829:i32, min value=w818:i32)  [unwired: 2 out]
                  n252 = case shown="True" w814 {
                    tunnel: w822 -> [_ w837]
                    tunnel: w808 -> [_ w836]
                    frame False {
                    }
                    frame True {
                      n253 = call-poly <userlib>:"Index Array Elements__ogtk.vi"("indices"=w836, "array"=w837) -> ("elements"=w838:dbl[])  [unwired: 9 in]
                      n254 = Index Array(array=w838) -> (element=w835:dbl)  [unwired: 1 in]
                      n255 = property on="Density (g/cc)" class="DigNum (strict)"("Value"=w835) -> ()  [unwired: 2 in, 2 out]
                    }
                  }
                  n256 = Increment(x=w829) -> (x+1=w825:i32)
                  n257 = Less Or Equal?(x=w812, y=w829) -> (x <= y?=w833:bool)
                  n258 = property on="New Type" class="DigNum (strict)"(error in=w830, "Maximum"=w825, "Minimum"=w818) -> (error out=w828:errorcluster)  [unwired: 1 in, 1 out]
                  n259 = Increment(x=w832) -> (x+1=w826:i32)
                  n260 = call-poly <userlib>:"Index Array Elements__ogtk.vi"("indices"=w809, "array"=w804) -> ("elements"=w806:i32[])  [unwired: 9 in]
                  n261 = property on="New Batch" class="DigNum (strict)"(error in=w828, "Maximum"=w826, "Minimum"=w817) -> (error out=w827:errorcluster)  [unwired: 1 in, 1 out]
                  n262 = Array Max & Min(array=w806) -> (max value=w807:i32)  [unwired: 3 out]
                  n263 = Increment(x=w807) -> (x+1=w805:i32)
                  n264 = case shown="True" w833 {
                    tunnel: w805 -> [_ w851]
                    tunnel: w827 -> [w841 w850]
                    tunnel: [w840 w849] -> w831
                    tunnel: w815 -> [w839 w848]
                    tunnel: w812 -> [_ w847]
                    tunnel: w808 -> [_ w846]
                    tunnel: w813 -> [_ w845]
                    tunnel: w820 -> [_ w844]
                    tunnel: w819 -> [_ w843]
                    frame False {
                      n265 = case shown="True" w839 {
                        frame False {
                        }
                        frame True {
                          n266 = invoke on="Typical Source Weight (g)" class="DigNum (strict)" method="Reinit To Default"() -> ()  [unwired: 3 in, 3 out]
                          n267 = invoke on="Size Range (diameter)" class="Str" method="Reinit To Default"() -> ()  [unwired: 3 in, 3 out]
                        }
                      }
                      n268 = property on="New Batch" class="DigNum (strict)"(error in=w841, "Value"=u16 1) -> (error out=w840:errorcluster)  [unwired: 1 in, 1 out]
                    }
                    frame True {
                      n269 = case shown="True" w848 {
                        tunnel: w847 -> [_ w861]
                        tunnel: w846 -> [_ w853]
                        tunnel: w845 -> [_ w862]
                        tunnel: w844 -> [_ w859]
                        tunnel: w843 -> [_ w858]
                        frame False {
                        }
                        frame True {
                          n270 = call-poly <userlib>:"Search Array__ogtk.vi"("Array"=w862, "Element Data"=w861) -> ("Indices of Elements"=w860:i32[])  [unwired: 7 in]
                          n271 = call-poly <userlib>:"Filter 1D Array__ogtk.vi"("items to filter"=w860, "array"=w853) -> ("filtered item indices"=w855:i32[])  [unwired: 4 in, 1 out]
                          n272 = Index Array(array=w855) -> (element=w854:i32)  [unwired: 1 in]
                          n273 = Index Array(array=w853, index=w854) -> (element=w852:i32)
                          n274 = Index Array(array=w858, index=w852) -> (element=w856:dbl)
                          n275 = Index Array(array=w859, index=w852) -> (element=w857:string)
                          n276 = property on="Typical Source Weight (g)" class="DigNum (strict)"("Value"=w856) -> ()  [unwired: 2 in, 2 out]
                          n277 = property on="Size Range (diameter)" class="Str"("Value"=w857) -> ()  [unwired: 2 in, 2 out]
                        }
                      }
                      n278 = property on="New Batch" class="DigNum (strict)"(error in=w850, "Value"=w851) -> (error out=w849:errorcluster)  [unwired: 1 in, 1 out]
                    }
                  }
                }
              }
              n279 = Not Equal?(x="", y=w775) -> (x != y?=w776:bool)
            }
            n280 = And(x=w703, y=w666) -> (x .and. y?=w667:bool)
            n281 = case shown="True" w667 {
              tunnel: w702 -> [w713 w772]
              tunnel: [w713 w772] -> w664
              tunnel: w700 -> [w712 w738]
              tunnel: [w712 w722] -> w699
              tunnel: w686 -> [_ w771]
              tunnel: w670 -> [_ w760]
              tunnel: w681 -> [_ w759]
              tunnel: w680 -> [_ w758]
              tunnel: w679 -> [_ w757]
              tunnel: w678 -> [_ w756]
              tunnel: w677 -> [_ w755]
              tunnel: w676 -> [_ w754]
              tunnel: w675 -> [_ w753]
              tunnel: w674 -> [_ w752]
              tunnel: w673 -> [_ w751]
              tunnel: w668 -> [_ w736]
              tunnel: w662 -> [_ w717]
              frame False {
              }
              frame True {
                n282 = Unbundle(w771) -> ("New Dust Name"=w770:string, "New Type"=w769:u16, "New Batch"=w768:u16, "dust type id"=w767:u16, "Dust Left (g)"=w766:dbl, "Typical Source Weight (g)"=w765:dbl, "Density (g/cc)"=w764:dbl, "Size Range (diameter)"=w763:string, "Comments"=w762:string, "Bottle Weight (g)"=w761:dbl, "Shoots"=w716:bool)
                n283 = Unbundle By Name(w771) -> ("New Dust Name"=w732:string, "New Type"=w731:u16, "New Batch"=w730:u16, "dust type id"=w733:u16, "Dust Left (g)"=w725:dbl, "Typical Source Weight (g)"=w728:dbl, "Density (g/cc)"=w729:dbl, "Size Range (diameter)"=w727:string, "Comments"=w724:string, "Bottle Weight (g)"=w726:dbl, "Shoots"=w714:bool)
                n284 = call <vilib>:"Trim Whitespace.vi"("string"=w770) -> ("trimmed string"=w719:string)  [unwired: 1 in]
                n285 = Build Array (concatenate)(w760, w719) -> (w741:string[])
                n286 = Build Array (concatenate)(w759, w769) -> (w750:i32[])
                n287 = Build Array (concatenate)(w758, w768) -> (w749:i32[])
                n288 = Build Array (concatenate)(w757, w767) -> (w748:i32[])
                n289 = Build Array (concatenate)(w756, w766) -> (w747:dbl[])
                n290 = Build Array (concatenate)(w755, w765) -> (w746:dbl[])
                n291 = Build Array (concatenate)(w717, w716) -> (w715:bool[])
                n292 = Build Array (concatenate)(w754, w764) -> (w745:dbl[])
                n293 = Build Array (concatenate)(w753, w763) -> (w744:string[])
                n294 = Build Array (concatenate)(w752, w762) -> (w743:string[])
                n295 = Build Array (concatenate)(w751, w761) -> (w742:dbl[])
                n296 = local write "Bottle Weights"(w742) -> ()
                n297 = call-poly <userlib>:"Remove Duplicates from 1D Array__ogtk.vi"("Input Array"=w741) -> ("Output Array"=w740:string[])  [unwired: 1 out]
                n298 = local write "Sizes"(w744) -> ()
                n299 = local write "Comments"(w743) -> ()
                n300 = local write "Densities"(w745) -> ()
                n301 = local write "Dust Weights"(w747) -> ()
                n302 = local write "Typical Weights"(w746) -> ()
                n303 = local write "Dust Type Ids"(w748) -> ()
                n304 = local write "Batch Nos"(w749) -> ()
                n305 = local write "Dust Names"(w741) -> ()
                n306 = local write "Dust Type"(w750) -> ()
                n307 = call <vilib>:"Trim Whitespace.vi"("string"=w732) -> ("trimmed string"=w718:string)  [unwired: 1 in]
                n308 = property on="Dust Name" class="CmbBox"("Strings[]"=w740) -> ()  [unwired: 2 in, 2 out]
                n309 = call <userlib>:"connect in.vi"("error in (no error)"=w738) -> ("error out"=w737:errorcluster, "Database Connection"=w739:T7)  [unwired: 7 in]
                n310 = Bundle("dust type id"=w733, "trimmed string"=w718, "New Type"=w731, "New Batch"=w730, "Density (g/cc)"=w729, "Typical Source Weight (g)"=w728, "Size Range (diameter)"=w727, "Bottle Weight (g)"=w726, "Dust Left (g)"=w725, "Comments"=w724, "Shoots"=w714) -> (w723:T13)  [unwired: 1 in]
                n311 = local write "Shoots"(w715) -> ()
                n312 = call <vilib>:"DB Tools Insert Data.vi"("data"=w723, "error in (no error)"=w737, "columns"=w736, "table"="dust_type", "connection reference"=w739) -> ("error out"=w721:errorcluster, "connection reference out"=w734:T7)  [unwired: 5 in]
                n313 = call <userlib>:"connect out.vi"("error in (no error)"=w737, "connection reference"=w734) -> ("error out"=w720:errorcluster)  [unwired: 9 in]
                n314 = Merge Errors(w721, w720) -> (w722:errorcluster)
              }
            }
            n315 = property on="Dust Name" class="CmbBox"(error in=w664) -> (error out=w663:errorcluster, "Value"=w665:string)  [unwired: 1 in, 1 out]
            n316 = property on="Update current entry" class="Bool (strict)"(error in=w664, "Visible"=w687, "Value"=w688) -> ()  [unwired: 1 in, 2 out]
            n317 = property on="Create New Entry" class="Bool (strict)"(error in=w664, "Visible"=w687, "Value"=w688) -> ()  [unwired: 1 in, 2 out]
            n318 = property on="Dust Properties" class="Clust (strict)"(error in=w664, "Visible"=w687) -> ()  [unwired: 1 in, 2 out]
            n319 = property on="New Dust" class="Clust (strict)"(error in=w664, "Visible"=w688) -> ()  [unwired: 1 in, 2 out]
            n320 = property on="Dust" class="Clust (strict)"(error in=w664, "Visible"=w687) -> ()  [unwired: 1 in, 2 out]
            n321 = property on="Update" class="Bool (strict)"(error in=w664, "Visible"=w688, "Value"=w688) -> ()  [unwired: 1 in, 2 out]
            n322 = property on="Cancel" class="Bool (strict)"(error in=w664, "Visible"=w688, "Value"=w688) -> ()  [unwired: 1 in, 2 out]
            n323 = property on="Dust Name" class="CmbBox"(error in=w663, "Val(Sgnl)"=w665) -> ()  [unwired: 1 in, 2 out]
          }
          event "Dust.Batch": Value Change {
            n324 = event-data() -> ()  [unwired: 1 in, 5 out]
            n325 = local read "Dust"() -> (w865:T4)
            n326 = Unbundle By Name(w865) -> ("Dust Name"=w864:string, "Type"=w877:u16, "Batch"=w875:u16)
            n327 = Equal?(x=w878, y=w877) -> (x = y?=w873:bool[])
            n328 = Equal?(x=w875, y=w876) -> (x = y?=w871:bool[])
            n329 = Equal?(x=w879, y=w864) -> (x = y?=w874:bool[])
            n330 = And(x=w874, y=w873) -> (x .and. y?=w872:bool[])
            n331 = And(x=w872, y=w871) -> (x .and. y?=w870:bool[])
            n332 = call-poly <userlib>:"Conditional Auto-Indexing Tunnel__ogtk.vi"("Array in"=w869, "Elements to keep"=w870) -> ("Filtered Array out"=w868:i32[])  [unwired: 5 in]
            n333 = Index Array(array=w868) -> (element=w867:i32)  [unwired: 1 in]
            n334 = property on="dust type id" class="Ring (strict)"(error in=w863, "Value"=w867) -> (error out=w866:errorcluster)  [unwired: 1 in, 1 out]
          }
          event "Dust.Type": Value Change {
            n335 = event-data() -> ()  [unwired: 1 in, 5 out]
            n336 = local read "Dust"() -> (w888:T4)
            n337 = Unbundle By Name(w888) -> ("Dust Name"=w887:string, "Type"=w898:u16, "Batch"=w897:u16)
            n338 = Equal?(x=w899, y=w898) -> (x = y?=w895:bool[])
            n339 = Equal?(x=w897, y=w883) -> (x = y?=w894:bool[])
            n340 = Equal?(x=w900, y=w887) -> (x = y?=w896:bool[])
            n341 = And(x=w896, y=w895) -> (x .and. y?=w884:bool[])
            n342 = call-poly <userlib>:"Conditional Auto-Indexing Tunnel__ogtk.vi"("Array in"=w883, "Elements to keep"=w884) -> ("Filtered Array out"=w882:i32[])  [unwired: 5 in]
            n343 = And(x=w884, y=w894) -> (x .and. y?=w893:bool[])
            n344 = Array Max & Min(array=w882) -> (max value=w880:i32, min value=w881:i32)  [unwired: 2 out]
            n345 = call-poly <userlib>:"Conditional Auto-Indexing Tunnel__ogtk.vi"("Array in"=w892, "Elements to keep"=w893) -> ("Filtered Array out"=w891:i32[])  [unwired: 5 in]
            n346 = property on="Batch" class="DigNum (strict)"(error in=w886, "Maximum"=w880, "Minimum"=w881) -> (error out=w885:errorcluster)  [unwired: 1 in, 1 out]
            n347 = Index Array(array=w891) -> (element=w890:i32)  [unwired: 1 in]
            n348 = property on="dust type id" class="Ring (strict)"(error in=w885, "Value"=w890) -> (error out=w889:errorcluster)  [unwired: 1 in, 1 out]
          }
        }
        n349 = case shown="No Error" w474 {
          selector: w474 -> [w491 _]
          tunnel: w474 -> [_ w494]
          frame No Error {
            n350 = case shown="True" "Clear Errors?" {
              tunnel: w491 -> [_ w493]
              frame False {
              }
              frame True {
                n351 = local write "error IO"(w493) -> ()
              }
            }
          }
          frame Error {
            n352 = local write "error IO"(w494) -> ()
          }
        }
        n353 = call <vilib>:"Clear Errors.vi"("error in (no error)"=w474) -> ("error out"=w479:errorcluster)  [unwired: 6 in]
      }
    }
    frame Error {
    }
  }
  "error IO" <- w60
